vi "FXP_AFMss_LinearDistEst_singleAxis.vi"() -> ()   [LabVIEW 2017]
uses:
  typeDefs/FXPControlParams_distEst.ctl
  fpga_fp_interface_lib/fpga_interface_types/boolean_indicators.ctl
  <vilib>/rvi/eio/common/nirviEmuClasses.ctl
  <vilib>/Platform/TimedLoop/XDataNode/timing_clust.ctl
  <vilib>/Platform/TimedLoop/XDataNode/nitl_modes.ctl
  <vilib>/Platform/TimedLoop/XDataNode/wakeup.ctl
  <vilib>/rvi/Emulation/niFpgaSctlEmulationGetInTimedLoop.vi
  <vilib>/rvi/Emulation/niFpgaProcessEmulError.vi
  <vilib>/rvi/eio/common/nirviEmuTemplateMethod_errors.vi
  <vilib>/rvi/Emulation/niFpgaGetClockAttributes.vi
  <vilib>/rvi/Emulation/niFpgaEmulationReportErrorSimple.vi
  <vilib>/rvi/Emulation/niFpgaCriticalErrorInLSC.vi
  <vilib>/rvi/Memory/Memory_Emulation/nirvimemoryFastEmulation.vi
  <vilib>/rvi/Memory/Memory_Emulation/nirvimemoryEmulation.vi
  <vilib>/rvi/Emulation/niFpgaEmulationIsFPGAContextNoSignature.vi
  <vilib>/rvi/DataTransferAndStorage/Container/Common/niFpgaContainerGetUniqueNameForEmu.vi
  <vilib>/rvi/errors/nirviReportUnexpectedCaseInternalError (U32).vi
  <vilib>/rvi/interface/RandomDataEmulation/niFpgaRandomDataHandleErrors.vi
  <vilib>/eio/EIOGrowableMethodNode/genericMethod/EIOGrowableMethodNode.xnode
  <vilib>/rvi/eio/nirviEIOMethodImplementation/nirviEIOMethodImplementation.xnode
  <vilib>/rvi/eio/nirviErrorMerge/nirviErrorMerge.xnode
  <vilib>/eio/EIONode/EIONode.xnode
  <vilib>/Platform/TimedLoop/XDataNode/XDataNode.xnode
  <vilib>/rvi/DataTransferAndStorage/Container/XNode/niFpgaContainer.xnode
  <vilib>/rvi/FXPMathLib/FxpSub/XNode/nifxpmath_Sub.xnode
  <vilib>/rvi/interface/RandomDataEmulation/nirviRandomDataFpgaReadWriteTemplate.vi
  <vilib>/Platform/TimedLoop/XDataNode/XDNodeRunTimeDep.lvlib
  <vilib>/rvi/FXPMathLib/sim/FxpSim.dll
panel:
  out "SS FIFO TimeOut?":bool
  out "u_k out":fxp<+/-,32,5>
  out "boolean  indicators":T1
  in  "du_umax":fxp<+/-,18,5>
  out "x-x(0)":fxp<+/-,18,5>
  in  "ControlParamsMpc":T2={"umax"=3.0, "NS"=0, "ref_f_VEC"=[0.0, 0.0], "Nu11_22"=[0.0, 0.0], "u0"=[0.0, 0.0]}
  out "y-axis fast":fxp<+/-,16,5>
  out "x(0)":fxp<+/-,16,5>
  out "LoopTicks2":u32
  out "Error Out":errorcluster
  out "x-axis fast":fxp<+/-,16,5>
  out "AI Timed Out":bool
  out "Stopped":bool
  in  "Settle Ticks":i16=1000
  in  "iters":i16=1
  in  "ymax":fxp<+/-,32,16>=4.0
  in  "TsTicks":i16
  out "Loop Ticks (benchmark)":i16
  out "NS":u8=2
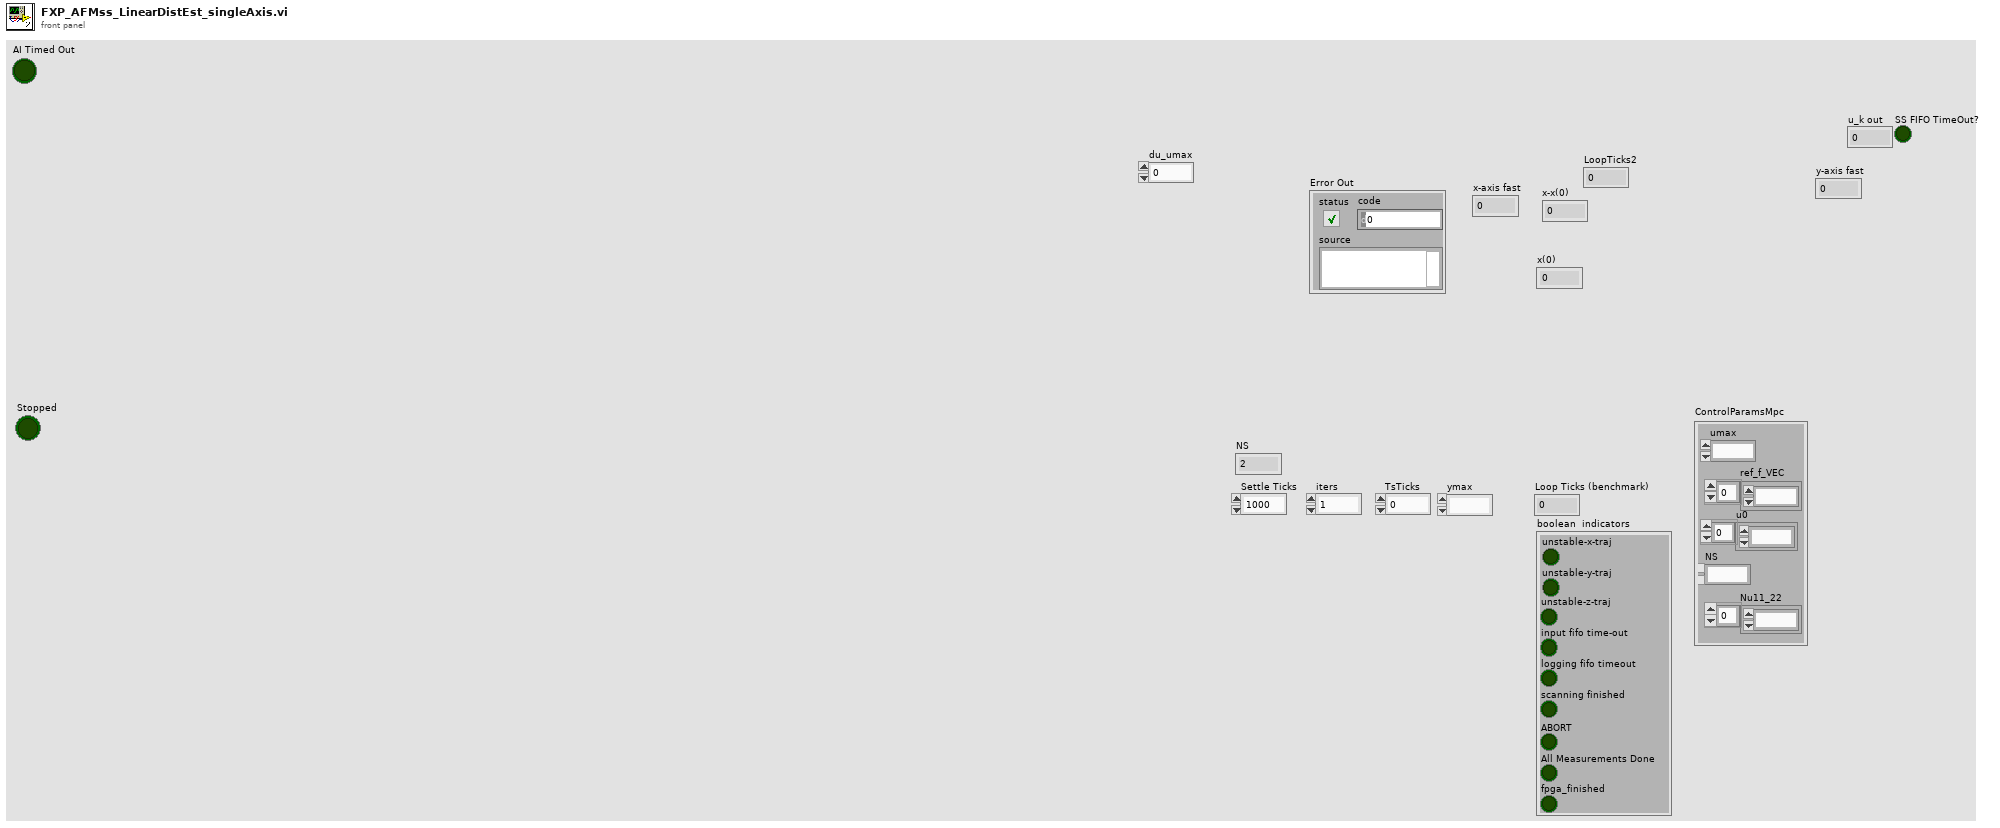
[diagram p1: front panel]
types:
  T1 = typedef "boolean_indicators.ctl" = cluster{"unstable-z-traj":bool, "input fifo time-out":bool, "logging fifo timeout":bool, "scanning finished":bool, "unstable-x-traj":bool, "unstable-y-traj":bool, "ABORT":bool, "All Measurements Done":bool, "fpga_finished":bool}
  T2 = typedef "FXPControlParams_distEst.ctl" = cluster{"umax":fxp<+/-,18,5>, "NS":u8, "ref_f_VEC":fxp<+/-,32,5>[], "Nu11_22":fxp<+/-,32,5>[], "u0":fxp<+/-,32,5>[]}
  T3 = typedef "nirviEmuClasses.ctl" = enum16{"IO Read", "IO Write", "Method", "Property Read", "Property Write"}
  T4 = typedef "XDNodeRunTimeDep.lvlib/timing_clust.ctl" = cluster{"Expected End [f-1]":u64, "Actual End [f-1]":u64, "Finished Late? [f-1]":bool, "Expected End [i-1]":u64, "Actual End [i-1]":u64, "Finished Late? [i-1]":bool, "Expected Start [i]":u64, "Actual Start [i]":u64, "Expected Start [f]":u64, "Actual Start [f]":u64, "Source Name":string, "Structure Name":string, "Period":i64, "Deadline":i64, "Offset":i64, "Start":i64, "Priority":i32, "Timeout":i32, "Mode":T5, "Wakeup Reason":T6, "Error":errorcluster, "Source Type":string, "Secondary Source Type":string, "Global End Time":u64, "Global Start Time":u64, "Frame Duration":u64, "Iteration Duration":u64, "Assigned CPU":i32, "I/O Scan Engine Mode":u32}
  T5 = typedef "XDNodeRunTimeDep.lvlib/nitl_modes.ctl" = enum32{"No Change", "Process missed periods, maintain original phase", "Discard missed periods, maintain original phase", "Process missed periods, ignore original phase", "Discard missed periods, ignore original phase"}
  T6 = typedef "XDNodeRunTimeDep.lvlib/wakeup.ctl" = enum32{"Normal", "Aborted", "Asynchronous wakeup", "Timing source error", "Timed loop error", "Timeout"}
  T7 = typedef "x_vec_type.ctl" = fxp<+/-,32,6>[]
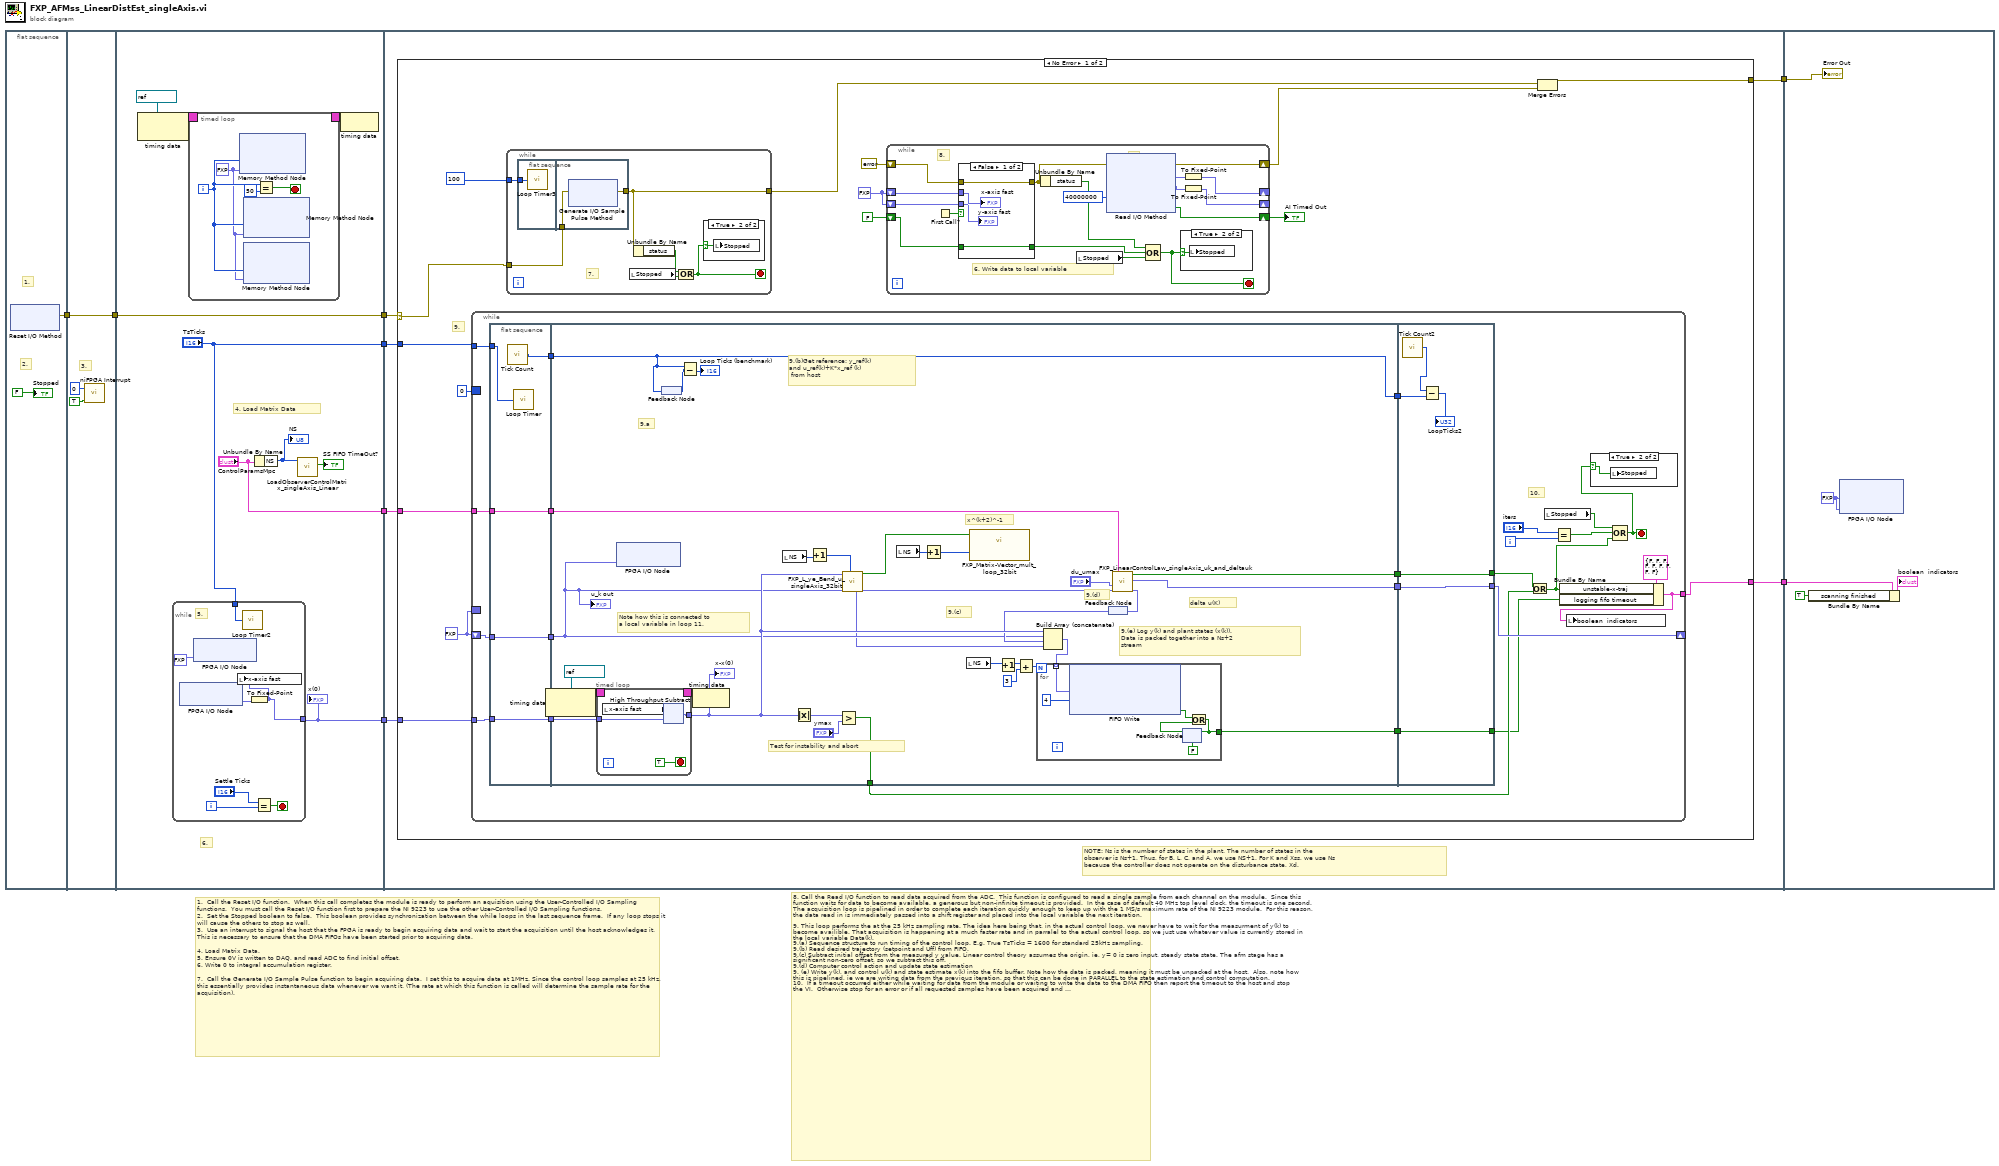
[diagram p0: block diagram]
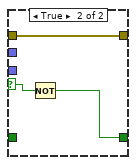
[diagram p2: hidden frame]
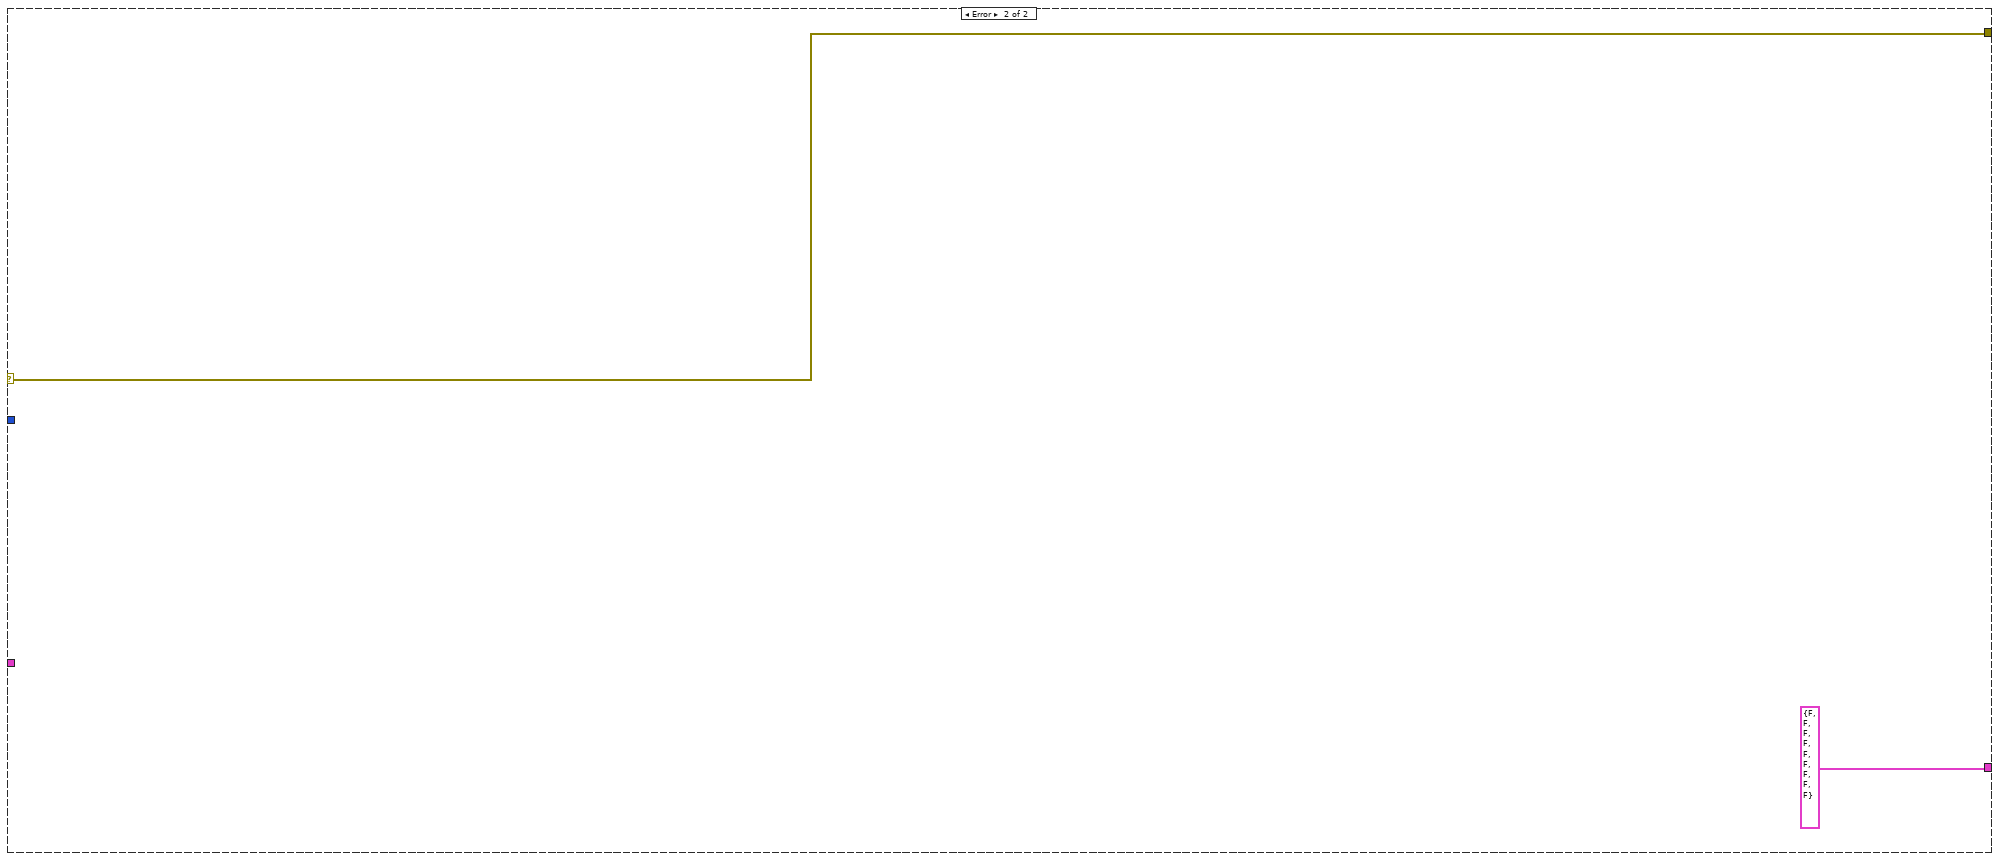
[diagram p6: hidden frame]
diagram:
  # "8. Call the Read I/O function to read data acquired from the ADC.  This function is configured to read a single sample from each channel on the module.  Since this function waits for data to become available, a generous but non-infinite timeout is provided.  In the case of default 40 MHz top level clock, the timeout is one second.  The acquisition loop is pipelined in order to complete each iteration quickly enough to keep up with the 1 MS/s maximum rate of the NI 9223 module.  For this reason, the data read in is immediately passed into a shift register and placed into the local variable the next iteration.\n\n9. This loop performs the at the 25 kHz sampling rate. The idea here being that, in the actual control loop, we never have to wait for the measurment of y(k) to become availible. That acquisition is happening at a much faster rate and in parralel to the actual control loop, so we just use whatever value is currently stored in the local variable Data(k).\n9.(a) Sequence structure to run timing of the control loop. E.g. True TsTicks = 1600 for standard 25kHz sampling.\n9.(b) Read desired trajectory (setpoint and Uff) from FIFO.\n9.(c) Subtract initial offset from the measured y value. Linear control theory assumes the origin, ie, y= 0 is zero input, steady state state. The afm stage has a significant non-zero offset, so we subtract this off.\n9.(d) Computer control action and update state estimation\n9. (e) Write y(k), and control u(k) and state estimate x(k) into the fifo buffer. Note how the data is packed, meaning it must be unpacked at the host.  Also, note how this is pipelined, ie we are writing data from the previous iteration, so that this can be done in PARALLEL to the state estimation and control computation.  \n10.  If a timeout occurred either while waiting for data from the module or waiting to write the data to the DMA FIFO then report the timeout to the host and stop the VI.  Otherwise stop for an error or if all requested samples have been acquired and placed into the DMA FIFO or if the controll law has detected instability.\n\n11. WRITE  TO DAQ. Note how the output of the control law is connected to loop 11 through a local variable."
  # "1.  Call the Reset I/O function.  When this call completes the module is ready to perform an aquisition using the User-Controlled I/O Sampling functions.  You must call the Reset I/O function first to prepare the NI 9223 to use the other User-Controlled I/O Sampling functions.\n2.  Set the Stopped boolean to false.  This boolean provides synchronization between the while loops in the last sequence frame.  If any loop stops it will cause the others to stop as well.\n3.  Use an interrupt to signal the host that the FPGA is ready to begin acquiring data and wait to start the acquisition until the host acknowledges it.  This is necessary to ensure that the DMA FIFOs have been started prior to acquiring data.\n\n4. Load Matrix Data.\n5. Ensure 0V is written to DAQ, and read ADC to find initial offset.\n6. Write 0 to integral accumulation register.\n\n7.  Call the Generate I/O Sample Pulse function to begin acquiring data.  I set this to acquire data at 1MHz. Since the control loop samples at 25 kHz, this essentially provides instantaneous data whenever we want it. (The rate at which this function is called will determine the sample rate for the acquisition)."
  n1 = flat-sequence {
    tunnel: [w9] -> w3
    tunnel: [w55] -> w4
    tunnel: w3 -> [w55]
    tunnel: ["TsTicks"] -> w8
    tunnel: [w66] -> w7
    tunnel: ["ControlParamsMpc"] -> w6
    tunnel: [w64] -> w5
    tunnel: w4 -> [w64]
    tunnel: w8 -> [w89]
    tunnel: w7 -> [w88]
    tunnel: w6 -> [w87]
    tunnel: w5 -> [w86]
    tunnel: [w85] -> w2
    tunnel: [w84] -> w1
    tunnel: w2 -> [w381]
    tunnel: w1 -> [w379]
    frame #0 {
      # "2."
      # "1."
      n2 = xnode "Reset I/O Method"() -> ("error out"=w9:errorcluster)  [unwired: 2 in, 1 out]
      "Stopped" <- FALSE ("Stopped")
    }
    frame #1 {
      # "3."
      n3 = call <vilib>:"niFPGA Interrupt.vi"("Wait Until Cleared (F)"=TRUE, "IRQ Number (0)"=u8 0) -> ()  [unwired: 1 in]
    }
    frame #2 {
      # "6."
      # "4. Load Matrix Data"
      n4 = node-c288(refnum<k21> "80MHz" ("Source Name")) -> (w63:T4)
      n5 = while {
        tunnel: [w81] -> w66
        tunnel: "TsTicks" -> [w83]
        i -> [w77]
        stop <- w79 stop-if-true
        # "5."
        n6 = xnode "FPGA I/O Node"() -> ("Mod2/AI0"=w82:fxp<+/-,24,5>)  [unwired: 1 in, 1 out]
        n7 = xnode "FPGA I/O Node"("Mod1/AO0"=fxp<+,1,1> 0.0) -> ()  [unwired: 1 in, 1 out]
        n8 = call "Loop Timer2"("Count(Ticks)"=w83) -> ()  [unwired: 1 out]
        n9 = To Fixed-Point(number=w82) -> (fixed-point=w81:fxp<+/-,16,5>)  [unwired: 1 in]
        n10 = local write "x-axis fast"(w81) -> ()
        n11 = Equal?(x="Settle Ticks", y=w77) -> (x = y?=w79:bool)
      }
      "x(0)" <- w66
      n12 = timed-loop {
        timing: w63 -> [_]
        timing-out: [_] -> w62
        i -> [w68]
        stop <- w70 stop-if-true
        w67 = fxp<+/-,32,5> 0.0 ("Data")
        n13 = xnode ("Memory Method Node")("Address"=w68, "Data"=w67) -> ()  [unwired: 1 in, 1 out]
        n14 = xnode ("Memory Method Node")("Address"=w68, "Data"=w67) -> ()  [unwired: 1 in, 1 out]
        n15 = xnode ("Memory Method Node")("Address"=w68, "Data"=w67) -> ()  [unwired: 1 in, 1 out]
        n16 = Equal?(x=w68, y=50) -> (x = y?=w70:bool)
      }
      n17 = Unbundle By Name("ControlParamsMpc") -> ("NS"=w59:u8)
      "NS" <- w59
      n18 = call "LoadObserverControlMatrix_singleAxis_Linear.vi"("NS"=w59) -> ("SS FIFO TimeOut?"=→"SS FIFO TimeOut?":bool)  [unwired: 10 in]
      n19 = node-c288(w62) -> ()
    }
    frame #3 {
      # "NOTE: Ns is the number of states in the plant. The number of states in the \nobserver is Ns+1. Thus, for B, L, C, and A, we use NS+1. For K and Xss, we use Ns\nbecause the controller does not operate on the disturbance state, Xd."
      n20 = case shown="No Error" w86 {
        selector: w86 -> [w93 w376]
        tunnel: w89 -> [w95 _]
        tunnel: w88 -> [w96 _]
        tunnel: w87 -> [w103 _]
        tunnel: [w100 w376] -> w85
        tunnel: [w91 T1 {"unstable-z-traj"=FALSE, "input fifo time-out"=FALSE, "logging fifo timeout"=FALSE, "scanning finished"=FALSE, "unstable-x-traj"=FALSE, "unstable-y-traj"=FALSE, "ABORT"=FALSE, "All Measurements Done"=FALSE, "fpga_finished"=FALSE} ("boolean  indicators 2")] -> w84
        frame No Error {
          w92 = fxp<+/-,18,5> 0.0
          w94 = fxp<+/-,16,5> 0.0 ("Mod1/AI0")
          # "9."
          n21 = while {
            border: i16 0 -> [_]
            tunnel: w103 -> [w313]
            shift-right: [w301] -> _
            shift-left: w92 -> [w311]
            tunnel: w96 -> [w310]
            tunnel: w95 -> [w302]
            border: w92 -> [_]
            tunnel: [w296] -> w91
            i -> [w314]
            stop <- w293 stop-if-true
            # "10."
            n22 = flat-sequence {
              tunnel: w310 -> [w319]
              tunnel: w311 -> [w320]
              tunnel: w313 -> [w321]
              tunnel: [w321] -> w306
              tunnel: [w320] -> w305
              tunnel: [w319] -> w304
              tunnel: [w318] -> w303
              tunnel: w302 -> [w317]
              tunnel: [w351] -> w297
              tunnel: [w331] -> w309
              tunnel: [w352] -> w308
              tunnel: [w350] -> w307
              tunnel: w303 -> [w350]
              tunnel: w304 -> [w341]
              tunnel: w305 -> [w328]
              tunnel: w306 -> [w338]
              tunnel: [w333] -> w300
              tunnel: [w374] -> w292
              tunnel: w309 -> [w370]
              tunnel: w308 -> [w374]
              tunnel: w307 -> [w372]
              tunnel: [w370] -> w301
              tunnel: [w369] -> w298
              tunnel: w300 -> [w369]
              frame #0 {
                n23 = call "Tick Count"() -> ("Tick Count(Ticks)"=w318:u32)
                n24 = call "Loop Timer"("Count(Ticks)"=w317) -> ()  [unwired: 1 out]
              }
              frame #1 {
                # "delta u(K)"
                # "Note how this is connected to\na local variable in loop 11."
                # "9.a"
                # "x^(k+2)^-1"
                # "9.(c)"
                # "9.(b)Get reference: y_ref(k)\nand u_ref(k)+K*x_ref (k)\n from host"
                # "9.(d)"
                # "9.(e) Log y(k) and plant states (x(k)). \nData is packed together into a Ns+2 \nstream"
                # "Test for instability and abort"
                n25 = node-c288(refnum<k21> "80MHz" ("Source Name")) -> (w345:T4)
                n26 = timed-loop {
                  timing: w345 -> [_]
                  timing-out: [_] -> w344
                  tunnel: w341 -> [w355]
                  tunnel: [w354] -> w332
                  stop <- TRUE stop-if-true
                  n27 = local read "x-axis fast"() -> (w356:fxp<+/-,16,5>)
                  n28 = xnode "High Throughput Subtract"("x"=w356, "y"=w355) -> ("x-y"=w354:fxp<+/-,18,5>)
                }
                "x-x(0)" <- w332
                n29 = xnode "FPGA I/O Node"("Mod1/AO0"=w328) -> ()  [unwired: 1 in, 1 out]
                n30 = feedback #1() -> (w342:u32)
                n31 = feedback-in #1(w350) -> ()
                n32 = Subtract(x=w350, y=w342) -> (x-y=→"Loop Ticks (benchmark)":u32)
                n33 = node-c288(w344) -> ()
                n34 = local read "NS"() -> (w346:u8)
                n35 = Absolute Value(x=w332) -> (abs(x)=w349:fxp<+,18,5>)
                n36 = Increment(x=w346) -> (x+1=w335:u8)
                n37 = Greater?(x=w349, y="ymax") -> (0:w351:bool)
                n38 = call "FXP_L_ye_Bend_u_singleAxis_32bit.vi"("NS"=w335, "U(k): ux"=w328, "Y(k): x"=w332) -> ("yd_est"=w336:fxp<+/-,32,5>, "outputValid"=w339:bool, "x0"=w322:T7)  [unwired: 6 in]
                n39 = local read "NS"() -> (w347:u8)
                n40 = Increment(x=w347) -> (x+1=w334:u8)
                n41 = local read "NS"() -> (w326:u8)
                n42 = call "FXP_Matrix-Vector_mult_loop_32bit.vi"("Ns_2"=w334, "inputValid"=w339) -> ()  [unwired: 9 in, 1 out]
                n43 = Increment(x=w326) -> (x+1=w325:u8)
                n44 = Add(x=w325, y=u8 3) -> (x+y=w323:u8)
                n45 = feedback #2() -> (w329:fxp<+/-,64,15>)
                n46 = Build Array (concatenate)(w332, w328, w329, w322) -> (w327:fxp<+/-,64,15>[])
                n47 = for {
                  N: w323 -> [_]
                  tunnel: w327 -> [w367] mode=indexing
                  tunnel: [w363] -> w352
                  n48 = xnode ("FIFO Write")("Element"=w367, "Timeout"=i16 4) -> ("Timed Out?"=w366:bool)  [unwired: 1 in, 1 out]
                  n49 = feedback #3(FALSE) -> (w365:bool)
                  n50 = Or(x=w366, y=w365) -> (x .or. y?=w363:bool)
                  n51 = feedback-in #3(w363) -> ()
                }
                n52 = call "FXP_LinearControlLaw_singleAxis_uk_and_deltauk.vi"("ControlParams_distEst"=w338, "yd_est_x"=w336, "du_max"="du_umax") -> ("del u_x"=w330:fxp<+/-,64,15>, "u_k (saturated)"=w331:fxp<+/-,32,5>, "saturated?"=w333:bool)  [unwired: 5 in, 1 out]
                n53 = feedback-in #2(w330) -> ()
                "u_k out" <- w328
              }
              frame #2 {
                n54 = call "Tick Count2"() -> ("Tick Count(Ticks)"=w373:u32)
                n55 = Subtract(x=w373, y=w372) -> (x-y=→"LoopTicks2":u32)
              }
            }
            n56 = Or(x=w298, y=w297) -> (x .or. y?=w294:bool)
            n57 = local read "Stopped"() -> (w295:bool)
            n58 = Equal?(x="iters", y=w314) -> (x = y?=w312:bool)
            n59 = Bundle By Name(cluster=T1 {"unstable-z-traj"=FALSE, "input fifo time-out"=FALSE, "logging fifo timeout"=FALSE, "scanning finished"=FALSE, "unstable-x-traj"=FALSE, "unstable-y-traj"=FALSE, "ABORT"=FALSE, "All Measurements Done"=FALSE, "fpga_finished"=FALSE} ("boolean  indicators"), "unstable-x-traj"=w294, "logging fifo timeout"=w292) -> (w296:T1)
            n60 = local write "boolean  indicators"(w296) -> ()
            n61 = Compound Arithmetic op=OR(w295, w312, w294) -> (w293:bool)
            n62 = case shown="True" w293 {
              selector: w293 -> [_ w316]
              frame False {
              }
              frame True {
                n63 = local write "Stopped"(w316) -> ()
              }
            }
          }
          n64 = while {
            tunnel: u32 100 ("Max TsTicks") -> [w243]
            tunnel: [w240] -> w98
            tunnel: w93 -> [w238]
            stop <- w239 stop-if-true
            # "7."
            n65 = flat-sequence {
              tunnel: w243 -> [w245]
              tunnel: [w247] -> w240
              tunnel: w238 -> [w246]
              frame #0 {
                n66 = call "Loop Timer3"("Count(Ticks)"=w245) -> ()  [unwired: 1 out]
              }
              frame #1 {
                n67 = xnode "Generate I/O Sample Pulse Method"("error in"=w246) -> ("error out"=w247:errorcluster)  [unwired: 1 in, 1 out]
              }
            }
            n68 = local read "Stopped"() -> (w242:bool)
            n69 = Unbundle By Name(w240) -> ("status"=w241:bool)
            n70 = Compound Arithmetic op=OR(w241, w242) -> (w239:bool)
            n71 = case shown="True" w239 {
              selector: w239 -> [_ w244]
              frame False {
              }
              frame True {
                n72 = local write "Stopped"(w244) -> ()
              }
            }
          }
          n73 = while {
            shift-right: [w120] -> w97
            shift-left: errorcluster {"status"=FALSE, "code"=0, "source"=""} ("error out") -> [w114]
            shift-right: [w119] -> w99
            shift-left: FALSE ("Timed Out") -> [w111]
            shift-right: [w109] -> _
            shift-left: w94 -> [w115]
            shift-right: [w107] -> _
            shift-left: w94 -> [w106]
            stop <- w118 stop-if-true
            # "8."
            # "6. Write data to local variable"
            # "5."
            n74 = First Call?() -> (First Call?: T/F=w112:bool)
            n75 = case shown="False" w112 {
              selector: w112 -> [_ w127]
              tunnel: [w123 w126] -> w116
              tunnel: w115 -> [w124 _]
              tunnel: w114 -> [w125 w128]
              tunnel: [w125 w128] -> w105
              tunnel: w111 -> [w123 _]
              tunnel: w106 -> [w122 _]
              frame False {
                "x-axis fast" <- w124
                "y-axis fast" <- w122
              }
              frame True {
                n76 = Not(x=w127) -> (.not. x?=w126:bool)
              }
            }
            n77 = Unbundle By Name(w105) -> ("status"=w113:bool)
            n78 = local read "Stopped"() -> (w117:bool)
            n79 = xnode "Read I/O Method"("error in"=w105, "Timeout"=40000000) -> ("error out"=w120:errorcluster, "Mod2/AI0"=w110:fxp<+/-,24,5>, "Mod2/AI1"=w108:fxp<+/-,24,5>, "Timed Out"=w119:bool)  [unwired: 2 in, 2 out]
            n80 = Compound Arithmetic op=OR(w113, w116, w117) -> (w118:bool)
            n81 = case shown="True" w118 {
              selector: w118 -> [_ w129]
              frame False {
              }
              frame True {
                n82 = local write "Stopped"(w129) -> ()
              }
            }
            n83 = To Fixed-Point(number=w110) -> (fixed-point=w109:fxp<+/-,16,5>)  [unwired: 1 in]
            n84 = To Fixed-Point(number=w108) -> (fixed-point=w107:fxp<+/-,16,5>)  [unwired: 1 in]
          }
          "AI Timed Out" <- w99
          n85 = Merge Errors(w98, w97) -> (w100:errorcluster)
        }
        frame Error {
        }
      }
    }
    frame #4 {
      w380 = fxp<+/-,20,5> 0.0 ("Mod1/AO0")
      n86 = Bundle By Name(cluster=w379, "scanning finished"=TRUE) -> (→"boolean  indicators":T1)
      n87 = xnode "FPGA I/O Node"("Mod1/AO0"=w380, "Mod1/AO1"=w380) -> ()  [unwired: 2 in, 2 out]
      "Error Out" <- w381
    }
  }
